vi "Create.vi"(11 "error in":errorcluster) -> (15 "error out":errorcluster)   [LabVIEW 2014, in "Error Logger.lvclass"]
uses:
  Error Logger.lvclass
  Error Logger.lvclass/Error Logger.ctl
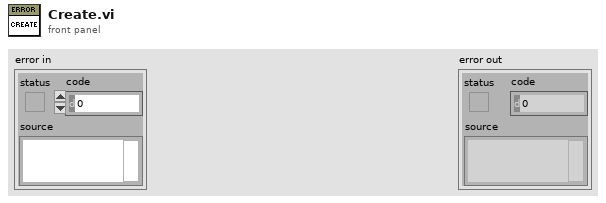
[diagram p1: front panel]
types:
  T1 = enum16{"open", "replace", "create", "open or create", "replace or create", "replace or create with confirmation"}
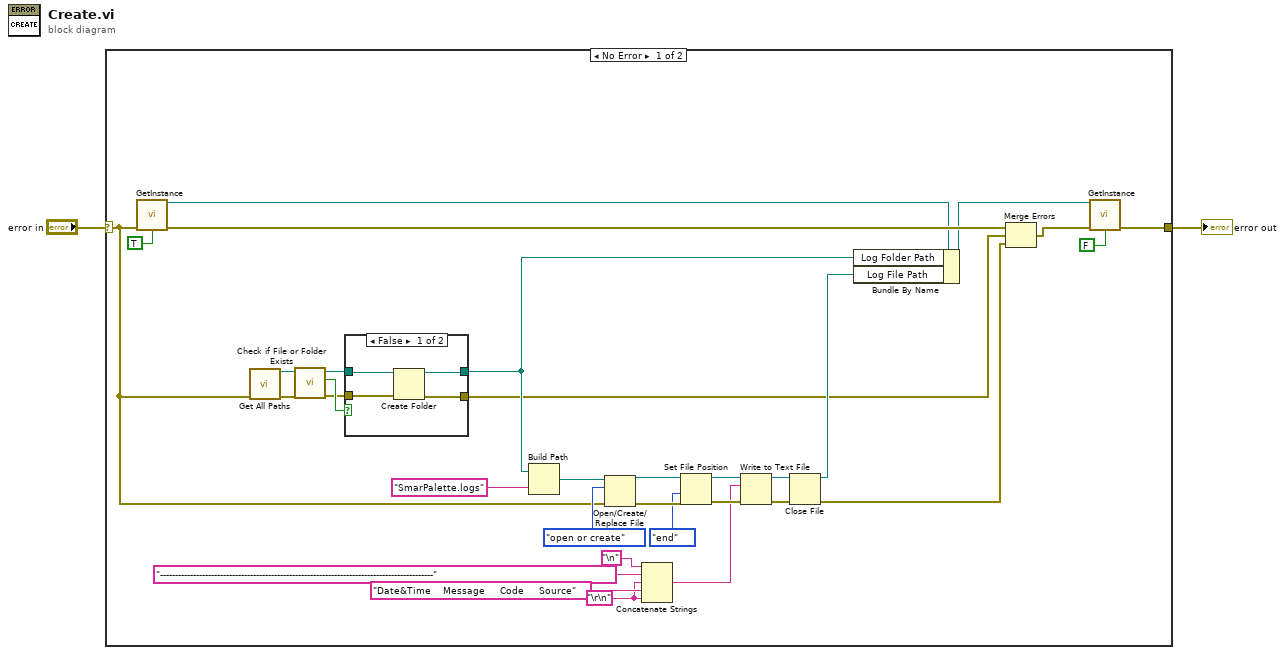
[diagram p0: block diagram]
diagram:
  n1 = case shown="No Error" "error in" {
    selector: "error in" -> [w11 w41]
    tunnel: [w8 w41] -> w1
    frame No Error {
      w5 = "\r\n"
      n2 = call "GetInstance.vi"("error in (no error)"=w11, "Get[T]\\Set[F]"=TRUE ("Get\\Set")) -> ("Error Logger out"=w33:refnum<class "Error Logger.lvclass">, "error out"=w34:errorcluster)  [unwired: 12 in]
      n3 = call "Get All Paths.vi"("error in"=w11) -> ("Log Folder"=w13:path, "error out"=w12:errorcluster)  [unwired: 9 in, 4 out]
      n4 = call <vilib>:"Check if File or Folder Exists.vi"("error in (no error)"=w12, "path"=w13) -> ("error out"=w29:errorcluster, "file or folder exists?"=w31:bool, "dup path"=w30:path)  [unwired: 7 in]
      n5 = case shown="False" w31 {
        tunnel: w30 -> [w38 w40]
        tunnel: [w37 w40] -> w28
        tunnel: w29 -> [w36 w39]
        tunnel: [w35 w39] -> w14
        frame False {
          n6 = Create Folder(path (use dialog)=w38, error in=w36) -> (created path=w37:path, error out=w35:errorcluster)  [unwired: 1 in, 1 out]
        }
        frame True {
        }
      }
      n7 = Build Path(base path=w28, name or relative path="SmarPalette.logs") -> (appended path=w27:path)
      n8 = Open/Create/Replace File(file path (use dialog)=w27, error in=w11, operation (0:open)=T1."open or create") -> (refnum out=w25:refnum<file>, error out=w24:errorcluster)  [unwired: 3 in, 1 out]
      n9 = Concatenate Strings("\n", "-------------------------------------------------------------------------------------------" ("string"), w5, "Date&Time    Message     Code     Source", w5) -> (w19:string)
      n10 = Set File Position(refnum=w25, from (0:start)=enum16{"start", "end", "current"}."end", error in=w24) -> (refnum out=w22:refnum<file>, error out=w21:errorcluster)  [unwired: 1 in]
      n11 = Write to Text File(file (use dialog)=w22, text=w19, error in=w21) -> (refnum out=w17:refnum<file>, error out=w18:errorcluster)  [unwired: 1 in, 1 out]
      n12 = Close File(refnum=w17, error in=w18) -> (path=w16:path, error out=w15:errorcluster)
      n13 = Bundle By Name(cluster=w33, "Log Folder Path"=w28, "Log File Path"=w16) -> (w7:refnum<class "Error Logger.lvclass">)
      n14 = Merge Errors(w34, w14, w15) -> (w9:errorcluster)
      n15 = call "GetInstance.vi"("Error Logger in"=w7, "error in (no error)"=w9, "Get[T]\\Set[F]"=FALSE ("Get\\Set")) -> ("error out"=w8:errorcluster)  [unwired: 11 in, 1 out]
    }
    frame Error {
    }
  }
  "error out" <- w1
